vi "host-C-1a.vi"() -> (0 "K(Indicator)":fxp<+/-,64,32>=1.52587890625e-05, 1 "degree":dbl=-171.37312679332166, 2 "Nominal Freq":fxp<+/-,64,32>=0.494873046875)   [LabVIEW 2012]
uses:
  <vilib>/FPGAPlugInAG/PCI-7831R/niLvFpga_Open_PCI-7831R.vi
  <vilib>/Utility/error.llb/Error Cluster From Error Code.vi
  <vilib>/rvi/errors/niLvFpgaAdjustHostInterfaceError.vi
  <vilib>/FPGAPlugInAG/PCI-7831R/niLvFpga_Abort_PCI-7831R.vi
  <vilib>/FPGAPlugInAG/PCI-7831R/niLvFpga_Close_PCI-7831R.vi
  <vilib>/rvi/interface/nirviOpenFPGA/nirviOpenFPGA.xnode
  SB130-XPS/Documents/FPGA-project-apporach-retraction/FPGA Bitfiles/Apporach-Retract_FPGATarget2_LIAFPGA3a1_LwIqbhm2wO0.lvbitx
  LIA_FPGA3a1.vi
  <vilib>/rvi/interface/nirviReadWriteControl/nirviReadWriteControl.xnode
  <vilib>/rvi/interface/nirviMethod/nirviMethod.xnode
  <vilib>/rvi/interface/nirviCloseFPGA/nirviCloseFPGA.xnode
  NiFpgaLv.dll
panel:
  out "VCO Sine Output":dbl(graph)
  out "VCO Frequency":dbl
  out "VCO Phase":dbl
  in  "Alpha (PID)":dbl=0.0010342
  in  "Phase Setpoint":dbl=1.57079632679
  out "Phase":dbl
  out "The Decs":dbl=7.8125e-09
  out "LSB Weight":dbl=0.00030517578125
  in  "K":fxp<+,16,0>=1.52587890625e-05
  in  "nominal freq 2":fxp<+,16,0>=0.494873046875
  out "x*y":dbl=0.015
  in  "stop 2":bool
  out "3rd stages":i32=1
  out "3rd decimation":i32=977
  out "1st decimation":i32=1
  out "2nd decimation":i32=128
  in  "Time Constant [s]":dbl=2.5 min=0.0 step=0.0001 format="%.2f"
  in  "Filter Rolloff":enum16{"20 dB", "40 dB", "60 dB", "80 dB"}(ring)
  out "Actual Sampling Frequency":dbl=200000.0
  in  "input range of 9205":dbl=10.0
  in  "Sampling Frequency":dbl=200000.0 min=1000.0 max=250000.0
  in  "stop":bool
  out "r":dbl(graph)=7.937638998845702e-07
  out "y":dbl=-1.1906385421752928e-07
  out "x":dbl=-7.84783363342285e-07
  out "f":dbl(graph)=94339.58418667316
  in  "dec2":i16=1
  in  "nominal freq":dbl=30000.0 min=500.0 max=125000.0
  in  "dec1":i16=1000
  in  "stages":i8=1 min=1 max=2
  in  "decimation":i16=1000
  # "Sampling Frequency"
  # "CIC First Decimation"
  # "CIC Second Decimation"
  # "MA Stages"
  # "MA Decimation"
  # "PLL Nominal Frequency"
  # "PLL Frequency Output"
  # "LIA Output"
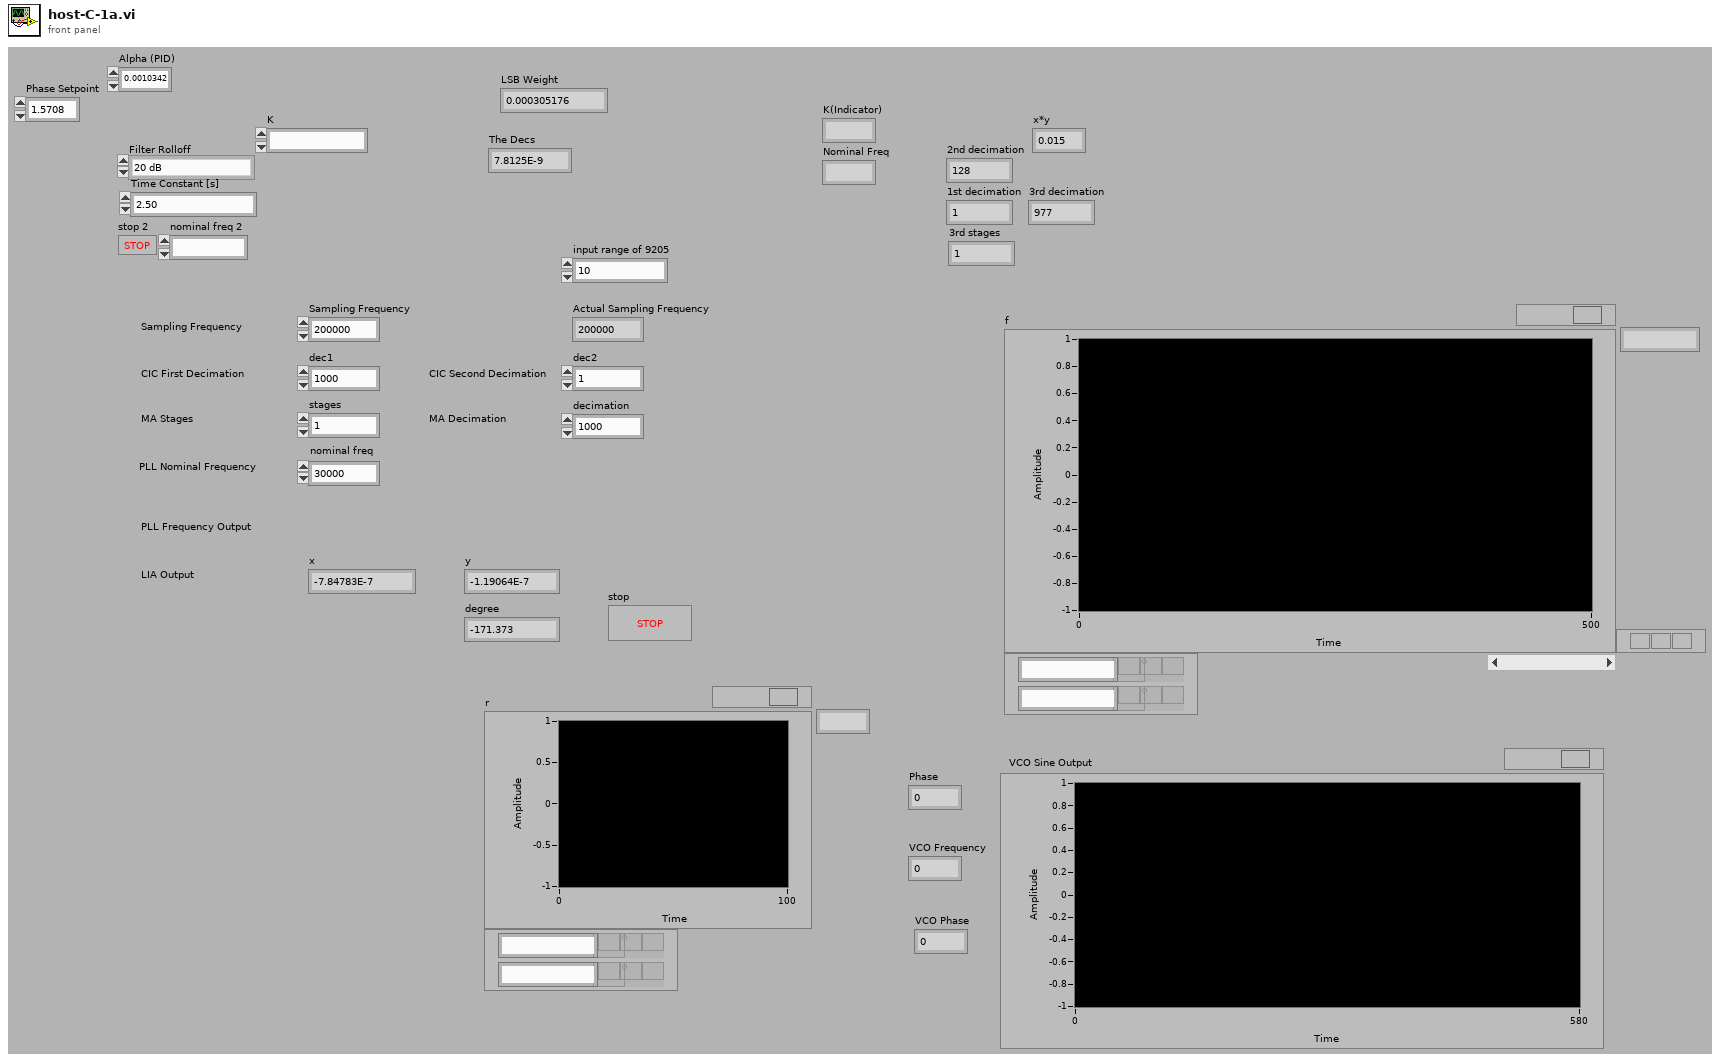
[diagram p1: front panel]
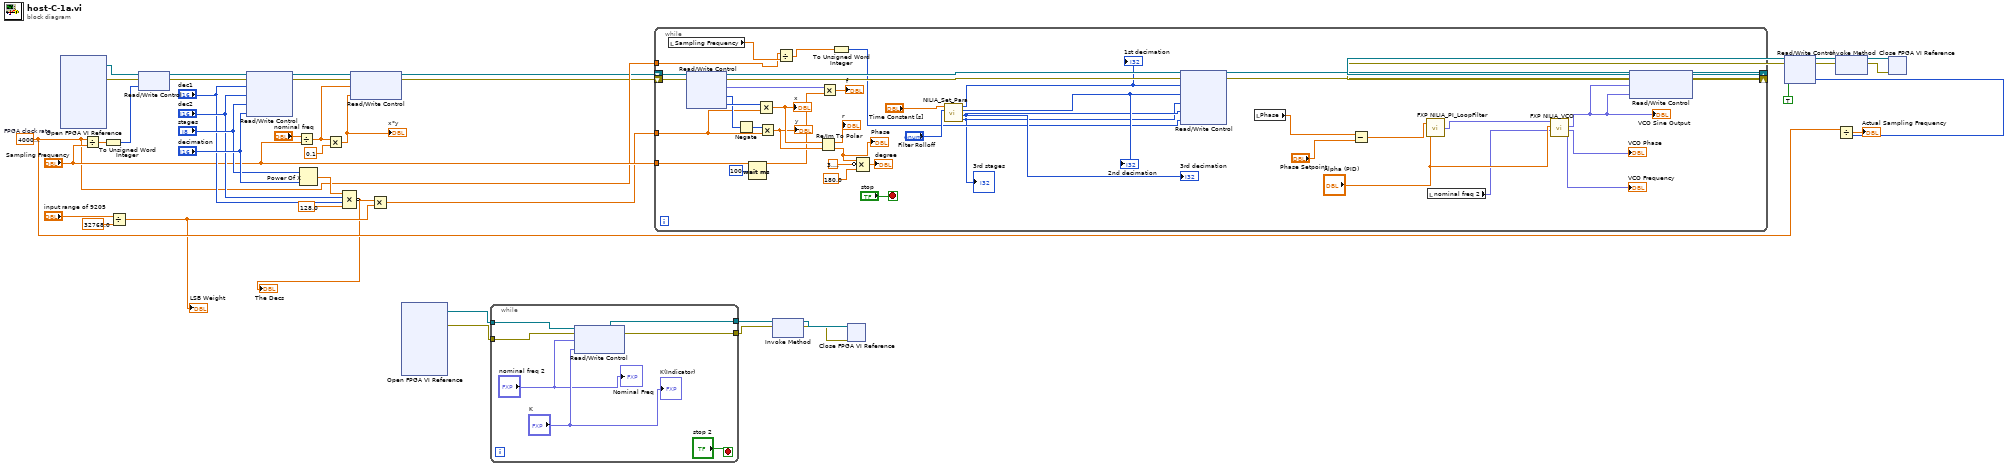
[diagram p0: block diagram]
diagram:
  w13 = 40000000.0  # FPGA clock rate
  n1 = xnode "Open FPGA VI Reference"() -> ("FPGA VI Reference Out"=w19:refnum<k20>, "error out"=w18:errorcluster)  [unwired: 2 in]
  n2 = Divide(x=w13, y="Sampling Frequency") -> (x/y=w25:dbl)
  n3 = To Unsigned Word Integer(number=w25) -> (unsigned 16bit integer=w24:u16)
  n4 = Divide(x="input range of 9205", y=32768.0) -> (x/y=w5:dbl)
  "LSB Weight" <- w5
  n5 = xnode "Read/Write Control"("FPGA VI Reference In"=w19, "error in"=w18, "Period"=w24) -> ("FPGA VI Reference Out"=w27:refnum<k20>, "error out"=w26:errorcluster)
  n6 = xnode "Read/Write Control"("FPGA VI Reference In"=w27, "error in"=w26, "dec1"="dec1", "dec2"="dec2", "stages"="stages", "decimation"="decimation") -> ("FPGA VI Reference Out"=w42:refnum<k20>, "error out"=w41:errorcluster)
  n7 = Divide(x="nominal freq", y="Sampling Frequency") -> (x/y=w21:dbl)
  n8 = Power Of X(1:"decimation", 2:"stages") -> (0:w38:dbl)
  n9 = Multiply(x=w21, y=0.1) -> (x*y=w6:dbl)
  "x*y" <- w6
  n10 = Compound Arithmetic op=MULTIPLY(w38, "dec2", "dec1", 128.0) -> (invert w4:dbl)
  "The Decs" <- w4
  n11 = xnode "Read/Write Control"("FPGA VI Reference In"=w42, "error in"=w41, "nominal freq"=w21, "K"=w6) -> ("FPGA VI Reference Out"=w2:refnum<k20>, "error out"=w1:errorcluster)
  n12 = Multiply(x=w4, y=w5) -> (x*y=w3:dbl)
  n13 = xnode "Open FPGA VI Reference"() -> ("FPGA VI Reference Out"=w12:refnum<k20>, "error out"=w11:errorcluster)  [unwired: 2 in]
  n14 = while {
    tunnel: w12 -> [w48]
    tunnel: w11 -> [w47]
    tunnel: [w46] -> w10
    tunnel: [w45] -> w9
    stop <- "stop 2" stop-if-true
    n15 = xnode "Read/Write Control"("FPGA VI Reference In"=w48, "error in"=w47, "nominal freq"="nominal freq 2", "K"="K") -> ("FPGA VI Reference Out"=w46:refnum<k20>, "error out"=w45:errorcluster)
    "K(Indicator)" <- "K"
    "Nominal Freq" <- "nominal freq 2"
  }
  n16 = while {
    shift-right: [w52] -> w34
    shift-left: w2 -> [w92]
    shift-right: [w51] -> w33
    shift-left: w1 -> [w91]
    tunnel: w3 -> [w88]
    tunnel: "Sampling Frequency" -> [w78]
    tunnel: w13 -> [w67]
    stop <- "stop" stop-if-true
    n17 = local read "Sampling Frequency"() -> (w68:dbl)
    n18 = xnode "Read/Write Control"("FPGA VI Reference In"=w92, "error in"=w91) -> ("FPGA VI Reference Out"=w75:refnum<k20>, "error out"=w74:errorcluster, "f"=w79:fxp<+/-,32,0>, "channelQ"=w89:i64, "channelI"=w90:i64)
    n19 = Negate(x=w89) -> (-x=w76:i64)
    n20 = Wait (ms)(milliseconds to wait=u32 100) -> ()  [unwired: 1 out]
    n21 = Multiply(x=w90, y=w88) -> (x*y=w87:dbl)
    "x" <- w87
    n22 = Multiply(x=w76, y=w88) -> (x*y=w86:dbl)
    "y" <- w86
    n23 = Divide(x=w67, y=w68) -> (x/y=w66:dbl)
    n24 = Re/Im To Polar(2:w86, 3:w87) -> (0:w63:dbl, 1:→"r":dbl)
    "Phase" <- w63
    n25 = Multiply(x=w79, y=w78) -> (x*y=→"f":dbl)
    n26 = To Unsigned Word Integer(number=w66) -> (unsigned 16bit integer=w65:u16)
    n27 = Compound Arithmetic op=MULTIPLY(w63, invert 3.141592653589793, 180.0 ("value")) -> (→"degree":dbl)
    n28 = call "NILIA_Set_Para.vi"("rolloff"="Filter Rolloff", "TC [sec]"="Time Constant [s]") -> ("3rd stages"=w64:i32, "3rd decimation"=w69:i32, "2nd decimation"=w70:i32, "1st decimation"=w71:i32)  [unwired: 5 in, 1 out]
    "2nd decimation" <- w70
    "1st decimation" <- w71
    "3rd decimation" <- w69
    "3rd stages" <- w64
    n29 = xnode "Read/Write Control"("FPGA VI Reference In"=w75, "error in"=w74, "dec1"=w71, "dec2"=w70, "stages"=w64, "decimation"=w69, "Period"=w65) -> ("FPGA VI Reference Out"=w54:refnum<k20>, "error out"=w53:errorcluster)
    n30 = local read "Phase"() -> (w62:dbl)
    n31 = Subtract(x=w62, y="Phase Setpoint") -> (x-y=w61:dbl)
    n32 = call "FXP NILIA_PI_LoopFilter.vi"("alpha [U16.-2]"="Alpha (PID)", "x [I16.2]"=w61) -> ("x+y [I32.17]"=w59:fxp<+/-,32,17>)  [unwired: 1 in]
    n33 = local read "nominal freq 2"() -> (w57:fxp<+,16,0>)
    n34 = call "FXP NILIA_VCO.vi"("nominal freq [U16.0]"=w57, "Kv [U16.0]"="Alpha (PID)", "v [I32.17]"=w59) -> ("f"=→"VCO Frequency":fxp<+/-,32,0>, "z [I32.1]"=→"VCO Phase":fxp<+/-,32,1>, "sin(z) [I16.2]"=w50:fxp<+/-,16,2>)  [unwired: 5 in, 1 out]
    "VCO Sine Output" <- w50
    n35 = xnode "Read/Write Control"("FPGA VI Reference In"=w54, "error in"=w53, "VCO Sinz Output"=w50, "Reference Signal"=w50) -> ("FPGA VI Reference Out"=w52:refnum<k20>, "error out"=w51:errorcluster)
  }
  n36 = xnode "Invoke Method"("FPGA VI Reference In"=w10, "error in"=w9) -> ("FPGA VI Reference Out"=w8:refnum<k20>, "error out"=w7:errorcluster)
  n37 = xnode "Close FPGA VI Reference"("FPGA VI Reference In"=w8, "error in"=w7) -> ()  [unwired: 1 out]
  n38 = xnode "Read/Write Control"("FPGA VI Reference In"=w34, "error in"=w33, "stop"=TRUE) -> ("FPGA VI Reference Out"=w31:refnum<k20>, "error out"=w30:errorcluster, "ticks"=w15:u16)
  n39 = xnode "Invoke Method"("FPGA VI Reference In"=w31, "error in"=w30) -> ("FPGA VI Reference Out"=w29:refnum<k20>, "error out"=w28:errorcluster)
  n40 = Divide(x=w13, y=w15) -> (x/y=→"Actual Sampling Frequency":dbl)
  n41 = xnode "Close FPGA VI Reference"("FPGA VI Reference In"=w29, "error in"=w28) -> ()  [unwired: 1 out]
